vi "5.10 Look Up Table.vi"(3 "Image Dst Out 2":T1, 4 "Output Buffer":T1, 5 "Input Fuzzy Blue Threshold":i32) -> (0 "Image Dst Out":T1, 1 "Lookup Table":u8[](array[numeric]), 2 "User Lookup":u8[](array[numeric])=[0, 20, 40])   [LabVIEW 2010]
uses:
  <vilib>/vision/Image Controls.llb/IMAQ Image.ctl
  <vilib>/gmath/statdist.llb/Normal CDF.vi
  <vilib>/vision/NI_Vision_Development_Module.lvlib
  <vilib>/gmath/NI_Gmath.lvlib
panel:
  in  "std":dbl=4.0
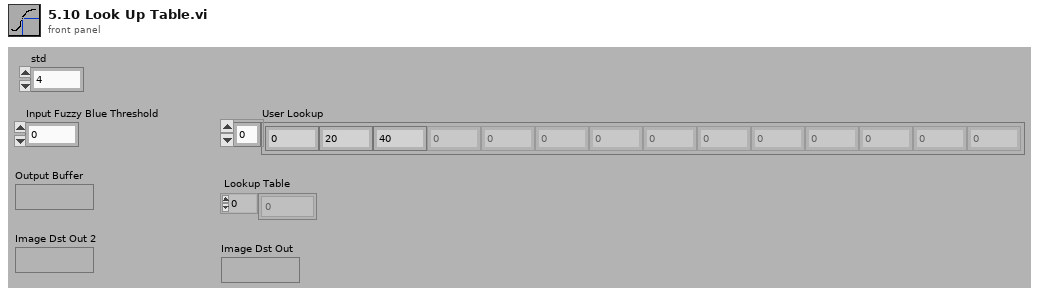
[diagram p1: front panel]
types:
  T1 = typedef "IMAQ Image.ctl" = refnum<image>
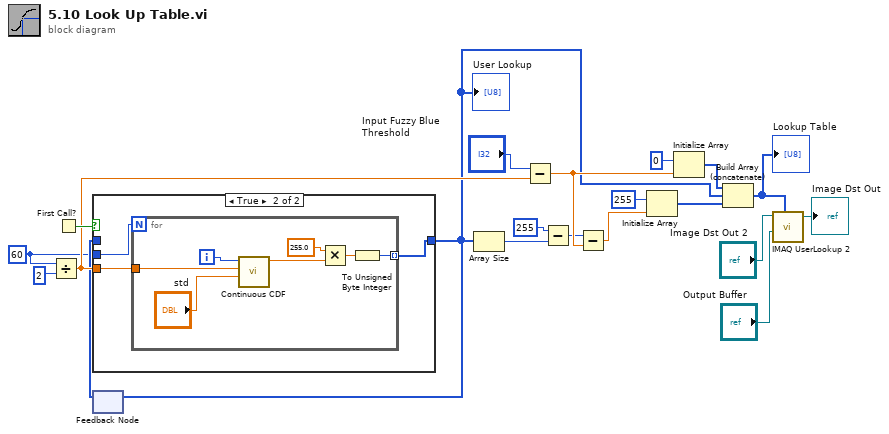
[diagram p0: block diagram]
diagram:
  w1 = 60
  n1 = Divide(x=w1, y=2 ("x")) -> (x/y=w19:dbl)
  n2 = First Call?() -> (First Call?: T/F=w20:bool)
  n3 = feedback #1() -> (w15:u8[])  [unwired: 1 in]
  n4 = case shown="True" w20 {
    tunnel: [w21 w24] -> w16
    tunnel: w15 -> [w21 _]
    tunnel: w19 -> [_ w23]
    tunnel: w1 -> [_ w22]
    frame False {
    }
    frame True {
      n5 = for {
        N: w22 -> [_]
        tunnel: [w26] -> w24 mode=indexing
        tunnel: w23 -> [w25]
        i -> [w31]
        n6 = call-poly <vilib>:"Continuous CDF.vi"("std"="std", "mean"=w25, "x"=w31) -> ("cdf(x)"=w29:dbl)  [unwired: 7 in, 1 out]
        n7 = Multiply(x=255.0, y=w29) -> (x*y=w27:dbl)
        n8 = To Unsigned Byte Integer(number=w27) -> (unsigned 8bit integer=w26:u8)
      }
    }
  }
  "User Lookup" <- w16
  n9 = feedback-in #1(w16) -> ()
  n10 = Array Size(array=w16) -> (size(s)=w9:i32)
  n11 = Subtract(x="Input Fuzzy Blue Threshold", y=w19) -> (x-y=w17:dbl)
  n12 = Subtract(x=u8 255, y=w9) -> (x-y=w10:i32)
  n13 = Subtract(x=w10, y=w17) -> (x-y=w12:dbl)
  n14 = Initialize Array(u8 255, w12) -> (w5:u8[])
  n15 = Initialize Array(u8 0, w17) -> (w4:u8[])
  n16 = Build Array (concatenate)(w4, w16, w5) -> (w13:u8[])
  "Lookup Table" <- w13
  n17 = call "IMAQ UserLookup 2"("Image Src"="Image Dst Out 2", "Lookup Table"=w13, "Image Dst"="Output Buffer") -> ("Image Dst Out"=→"Image Dst Out":T1)  [unwired: 4 in, 1 out]
